vi "TP04300 Poll Temperature.vi"() -> ()   [LabVIEW 2010]
doc: "Use this template to parse data acquired from an instrument attached to your computer through a GPIB, serial, or other port and write the data to a file. Note: VIs created from this template will have automatic error handling enabled by default."
uses:
  Temptronic TP04300.lvlib
panel:
  out "Air Flow":dbl format="%#.1g"
  out "TP04300 ID":string caption="Instrument Information"
  in  "Setpoint":dbl=25.0 caption="Enter \nSetpoint, C" min=-150.0 max=225.0 step=0.1 format="%.1f"
  in  "VISA resource name":refnum<visa-resource-name>
  in  "Start Flow":bool
  out "Temperature Graph":dbl[][](graph)
  in  "Stop":bool
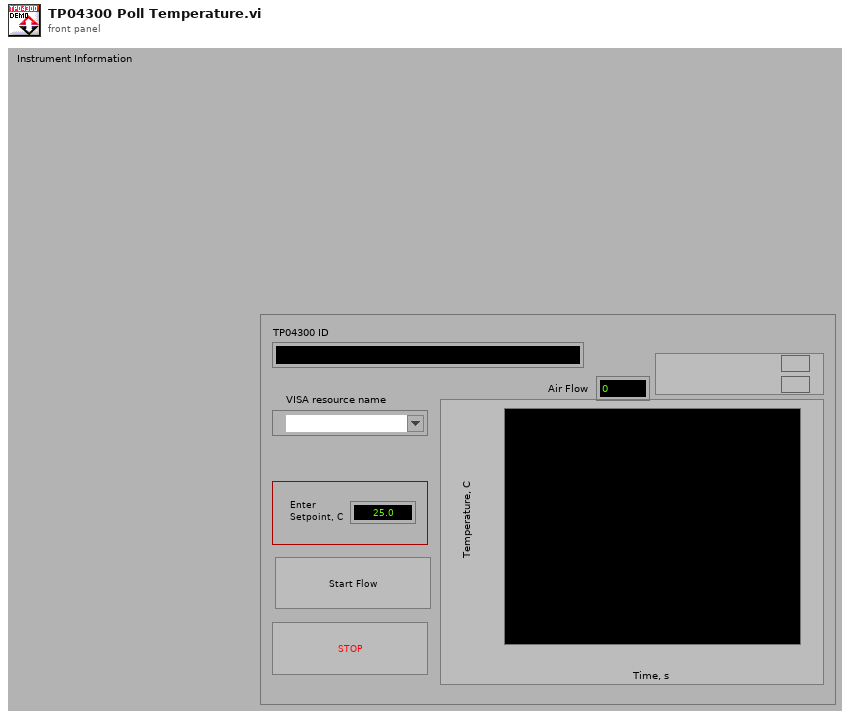
[diagram p1: front panel]
types:
  T1 = cluster{"Baud Rate":u32, "Parity":u16, "Data Bits":u16, "Stop Bits":u16, "Flow Control":u16}
  T2 = enum16{"Air Flow", "Trickle Flow", "Head", "Head Lock", "Compressor"}
  T3 = enum16{"Head Down & Air On", "Head Up & Air Off", "Air Flow Off", "Air Flow On", "Trickle Flow Off", "Trickle Flow On", "Head Up", "Head Down", "Head Lock Off", "Head Lock On", "Compressor Off", "Compressor On"}
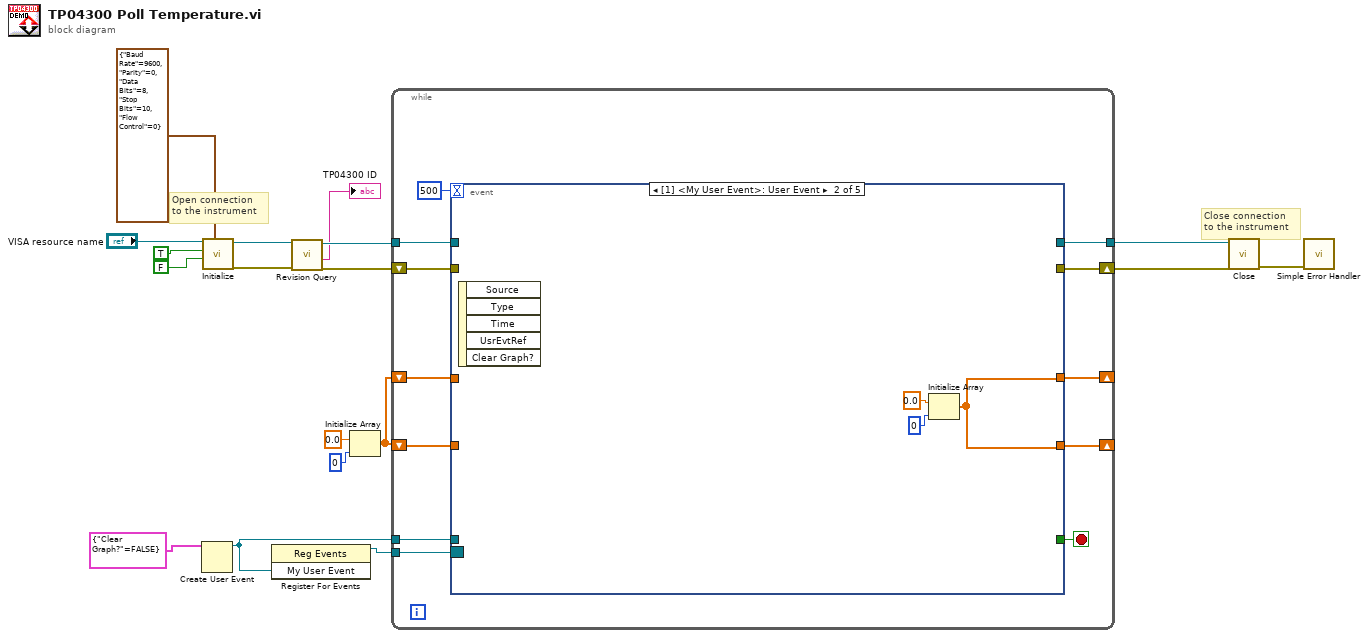
[diagram p0: block diagram]
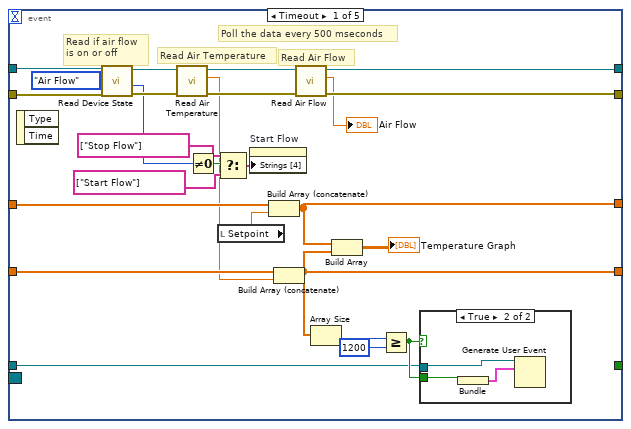
[diagram p2: hidden frame]
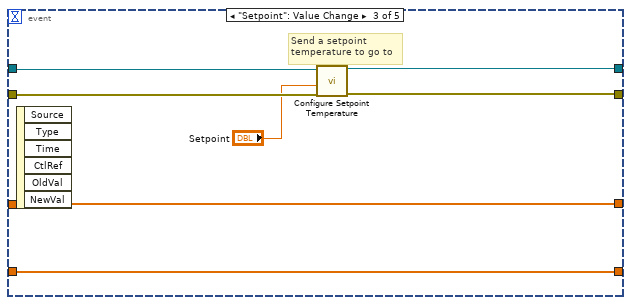
[diagram p4: hidden frame]
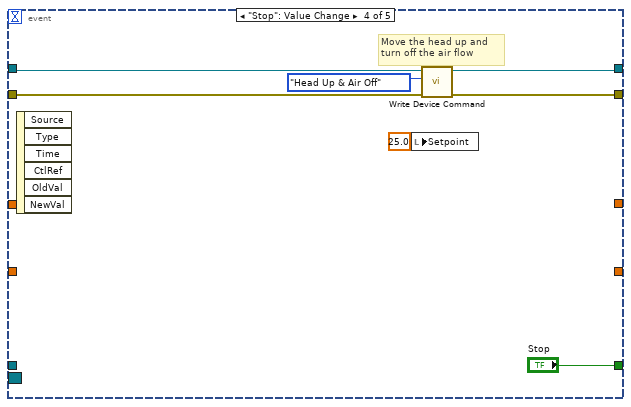
[diagram p5: hidden frame]
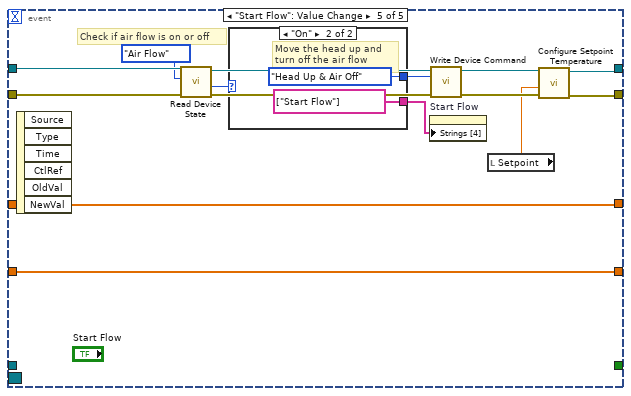
[diagram p6: hidden frame]
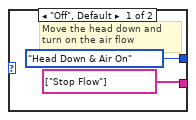
[diagram p7: hidden frame]
diagram:
  # "Open connection \nto the instrument"
  # "Close connection \nto the instrument"
  n1 = Create User Event(user event datatype=cluster{"Clear Graph?":bool} {"Clear Graph?"=FALSE} ("My User Event")) -> (user event=w10:refnum<user-event>)  [unwired: 1 in, 1 out]
  n2 = call "Initialize.vi"("Serial Configuration"=T1 {"Baud Rate"=9600, "Parity"=0, "Data Bits"=8, "Stop Bits"=10, "Flow Control"=0}, "Reset (True)"=FALSE ("ID Query? (T: Yes)"), "ID Query (True)"=TRUE ("ID Query? (T: Yes)"), "VISA resource name"="VISA resource name") -> ("error out"=w5:errorcluster, "VISA resource name out"=w8:refnum<visa-resource-name>)  [unwired: 6 in]
  n3 = register-events(w10) -> (reference out=w12:refnum<event-registration>)  [unwired: 2 in, 1 out]
  n4 = call "Revision Query.vi"("error in (no error)"=w5, "VISA resource name"=w8) -> ("error out"=w6:errorcluster, "Instrument Information"=→"TP04300 ID":string, "VISA resource name out"=w7:refnum<visa-resource-name>)  [unwired: 6 in, 1 out]
  n5 = Initialize Array(0.0 ("element"), 0 ("dimension size")) -> (w13:dbl[])
  n6 = while {
    tunnel: w7 -> [w29]
    tunnel: [w28] -> w3
    shift-right: [w26] -> w2
    shift-left: w6 -> [w27]
    shift-right: [w23] -> _
    shift-left: w13 -> [w24]
    shift-right: [w21] -> _
    shift-left: w13 -> [w22]
    tunnel: w12 -> [w20]
    tunnel: w10 -> [w19]
    stop <- w30 stop-if-true
    n7 = event shown="[1] <My User Event>: User Event" {
      selector: w20 -> [_ _ _ _ _]
      dyn-events: _ -> [_ _ _ _ _]
      timeout: 500 -> [_ _ _ _ _]
      tunnel: [_ _ _ "Stop" _] -> w30
      tunnel: w29 -> [w51 _ w65 w72 w90]
      tunnel: [w53 _ w66 w71 w78] -> w28
      tunnel: w27 -> [w49 _ w68 w75 w91]
      tunnel: [w55 _ w67 w74 w80] -> w26
      tunnel: w24 -> [w37 _ w69 _ w83]
      tunnel: [w35 w60 w69 _ w83] -> w23
      tunnel: w22 -> [w39 _ w63 _ w82]
      tunnel: [w41 w60 w63 _ w82] -> w21
      tunnel: w19 -> [w31 _ _ _ _]
      event Timeout {
        # "Read if air flow \nis on or off"
        # "Read Air Temperature"
        # "Read Air Flow"
        # "Poll the data every 500 mseconds"
        n8 = event-data() -> ()  [unwired: 1 in, 2 out]
        n9 = call "Read Device State.vi"("error in (no error)"=w49, "Device Command"=T2."Air Flow", "VISA resource name"=w51) -> ("error out"=w48:errorcluster, "Device Reply"=w42:enum16{"Off", "On"}, "VISA resource name out"=w50:refnum<visa-resource-name>)  [unwired: 5 in, 1 out]
        n10 = call "Read Air Temperature.vi"("error in (no error)"=w48, "VISA resource name"=w50) -> ("error out"=w56:errorcluster, "Air Temperature"=w36:dbl, "VISA resource name out"=w54:refnum<visa-resource-name>)  [unwired: 7 in]
        n11 = Not Equal To 0?(x=w42) -> (x != 0?=w46:bool)
        n12 = Select(t=string[] ["Stop Flow"] ("Strings [4]"), s=w46, f=string[] ["Start Flow"] ("Strings [4]")) -> (s? t:f=w43:string[])
        n13 = local read "Setpoint"() -> (w38:dbl)
        n14 = property on="Start Flow" class="Bool"("Strings [4]"=w43) -> ()  [unwired: 2 in, 2 out]
        n15 = Build Array (concatenate)(w39, w38) -> (w41:dbl[])
        n16 = Build Array (concatenate)(w37, w36) -> (w35:dbl[])
        n17 = call "Read Air Flow.vi"("error in (no error)"=w56, "VISA resource name"=w54) -> ("error out"=w55:errorcluster, "Air Flow"=→"Air Flow":dbl, "VISA resource name out"=w53:refnum<visa-resource-name>)  [unwired: 6 in, 1 out]
        n18 = Array Size(array=w35) -> (size(s)=w34:i32)
        n19 = Build Array(w41, w35) -> (→"Temperature Graph":dbl[][])
        n20 = Greater Or Equal?(x=w34, y=1200) -> (x >= y?=w32:bool)
        n21 = case shown="True" w32 {
          tunnel: w31 -> [_ w59]
          tunnel: w32 -> [_ w58]
          frame False {
          }
          frame True {
            n22 = Bundle(w58) -> (w57:cluster{bool})  [unwired: 1 in]
            n23 = Generate User Event(user event=w59, event data cluster=w57) -> ()  [unwired: 1 in, 2 out]
          }
        }
      }
      event User Event {
        n24 = event-data() -> ()  [unwired: 1 in, 5 out]
        n25 = Initialize Array(0.0 ("element"), 0 ("dimension size")) -> (w60:dbl[])
      }
      event "Setpoint": Value Change {
        # "Send a setpoint \ntemperature to go to"
        n26 = event-data() -> ()  [unwired: 1 in, 6 out]
        n27 = call "Configure Setpoint Temperature.vi"("error in (no error)"=w68, "Setpoint (0)"="Setpoint", "VISA resource name"=w65) -> ("error out"=w67:errorcluster, "VISA resource name out"=w66:refnum<visa-resource-name>)  [unwired: 7 in]
      }
      event "Stop": Value Change {
        # "Move the head up and \nturn off the air flow"
        n28 = event-data() -> ()  [unwired: 1 in, 6 out]
        n29 = local write "Setpoint"(25.0 ("Setpoint")) -> ()
        n30 = call "Write Device Command.vi"("error in (no error)"=w75, "Device Command"=T3."Head Up & Air Off", "VISA resource name"=w72) -> ("error out"=w74:errorcluster, "VISA resource name out"=w71:refnum<visa-resource-name>)  [unwired: 7 in]
      }
      event "Start Flow": Value Change {
        # "Check if air flow is on or off"
        n31 = event-data() -> ()  [unwired: 1 in, 6 out]
        n32 = call "Read Device State.vi"("error in (no error)"=w91, "Device Command"=T2."Air Flow", "VISA resource name"=w90) -> ("error out"=w87:errorcluster, "Device Reply"=w88:enum16{"Off", "On"}, "VISA resource name out"=w86:refnum<visa-resource-name>)  [unwired: 5 in, 1 out]
        n33 = case shown="\"On\"" w88 {
          tunnel: [T3."Head Down & Air On" ("Device Command") T3."Head Up & Air Off" ("Device Command")] -> w85
          tunnel: [string[] ["Stop Flow"] ("Strings [4]") string[] ["Start Flow"] ("Strings [4]")] -> w84
          frame "Off", Default {
            # "Move the head down and \nturn on the air flow"
          }
          frame "On" {
            # "Move the head up and \nturn off the air flow"
          }
        }
        n34 = property on="Start Flow" class="Bool"("Strings [4]"=w84) -> ()  [unwired: 2 in, 2 out]
        n35 = call "Write Device Command.vi"("error in (no error)"=w87, "Device Command"=w85, "VISA resource name"=w86) -> ("error out"=w81:errorcluster, "VISA resource name out"=w79:refnum<visa-resource-name>)  [unwired: 7 in]
        n36 = local read "Setpoint"() -> (w77:dbl)
        n37 = call "Configure Setpoint Temperature.vi"("error in (no error)"=w81, "Setpoint (0)"=w77, "VISA resource name"=w79) -> ("error out"=w80:errorcluster, "VISA resource name out"=w78:refnum<visa-resource-name>)  [unwired: 7 in]
      }
    }
  }
  n38 = call "Close.vi"("error in (no error)"=w2, "VISA resource name"=w3) -> ("error out"=w9:errorcluster)  [unwired: 9 in]
  n39 = call <vilib>:"Simple Error Handler.vi"("error in (no error)"=w9) -> ()  [unwired: 4 in, 5 out]
